vi "4 ch 8or12kHz resonance scanner (FPGA) fixed pix clock.vi"() -> ()   [LabVIEW 2012]
uses:
  <vilib>/eio/EIONode/EIONode.xnode
  <vilib>/rvi/eio/common/nirviEmuTemplateMethod_errors.vi
  <vilib>/rvi/DataTransferAndStorage/Container/XNode/niFpgaContainer.xnode
  <vilib>/platform/TimedLoop/XDataNode/XDataNode.xnode
  <vilib>/Platform/TimedLoop/XDataNode/nitl_modes.ctl
  <vilib>/Platform/TimedLoop/XDataNode/XDNodeRunTimeDep.lvlib
  <vilib>/Platform/TimedLoop/XDataNode/wakeup.ctl
  <vilib>/Platform/TimedLoop/XDataNode/timing_clust.ctl
  <vilib>/rvi/interface/RandomDataEmulation/nirviRandomDataFpgaReadWriteTemplate.vi
panel:
  in  "frequency (T:8kHz F:12kHz)":bool
  in  "lines at once":i16=4999
  in  "Start Delay (Ticks)":i16 caption="Start delay (Ticks)"
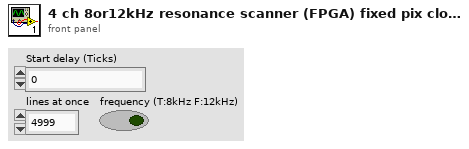
[diagram p1: front panel]
types:
  T1 = typedef "XDNodeRunTimeDep.lvlib/timing_clust.ctl" = cluster{"Expected End [f-1]":u64, "Actual End [f-1]":u64, "Finished Late? [f-1]":bool, "Expected End [i-1]":u64, "Actual End [i-1]":u64, "Finished Late? [i-1]":bool, "Expected Start [i]":u64, "Actual Start [i]":u64, "Expected Start [f]":u64, "Actual Start [f]":u64, "Source Name":string, "Structure Name":string, "Period":i64, "Deadline":i64, "Offset":i64, "Start":i64, "Priority":i32, "Timeout":i32, "Mode":T2, "Wakeup Reason":T3, "Error":errorcluster, "Source Type":string, "Secondary Source Type":string, "Global End Time":u64, "Global Start Time":u64, "Frame Duration":u64, "Iteration Duration":u64, "Assigned CPU":i32, "I/O Scan Engine Mode":u32}
  T2 = typedef "XDNodeRunTimeDep.lvlib/nitl_modes.ctl" = enum32{"No Change", "Process missed periods, maintain original phase", "Discard missed periods, maintain original phase", "Process missed periods, ignore original phase", "Discard missed periods, ignore original phase"}
  T3 = typedef "XDNodeRunTimeDep.lvlib/wakeup.ctl" = enum32{"Normal", "Aborted", "Asynchronous wakeup", "Timing source error", "Timed loop error", "Timeout"}
  T4 = cluster{"IO Module\\AI A0":i32, "IO Module\\AI A1":i32, "IO Module\\AI A3":i32, "IO Module\\AI A6":i32, "IO Module\\AI B8":i32}
  T5 = cluster{"IO Module\\AI A0":i16, "IO Module\\AI A1":i16, "IO Module\\AI A3":i16, "IO Module\\AI A6":i16, "IO Module\\AI B8":i16}
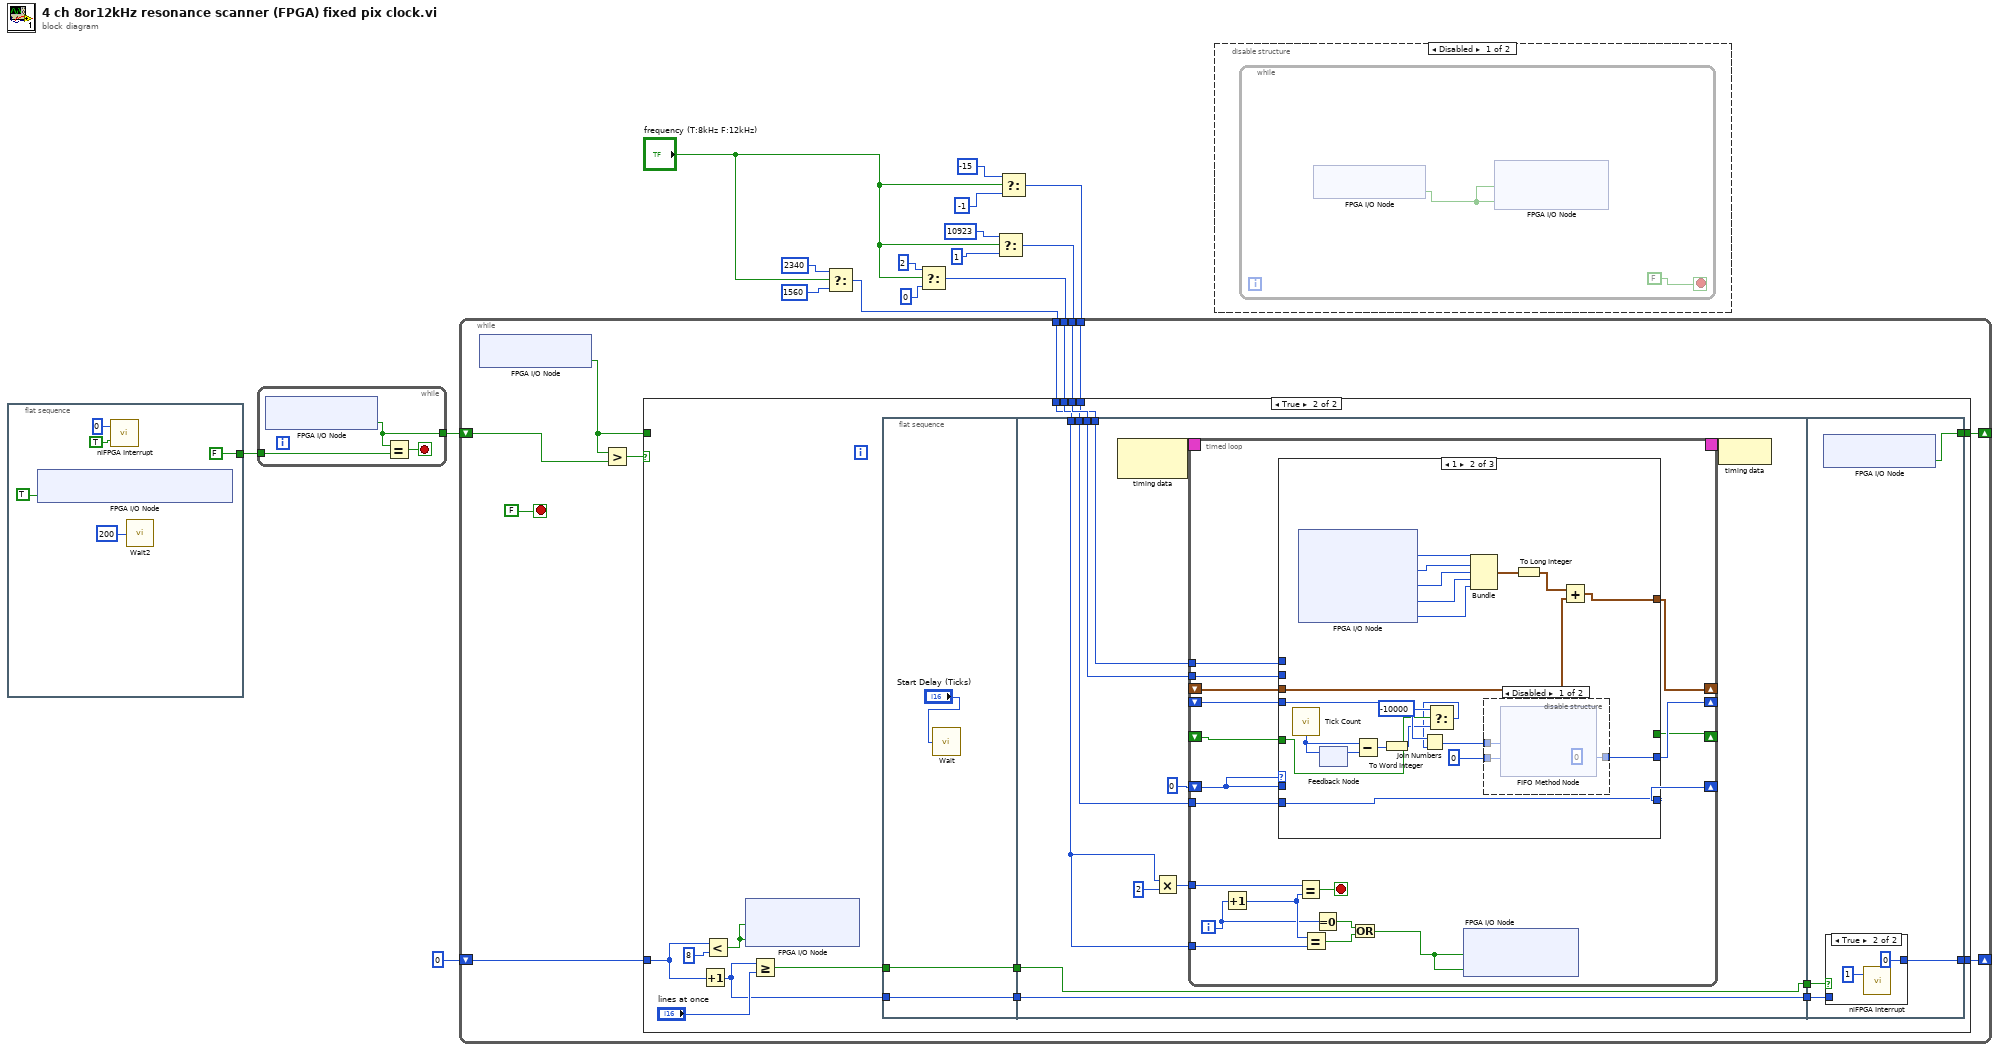
[diagram p0: block diagram]
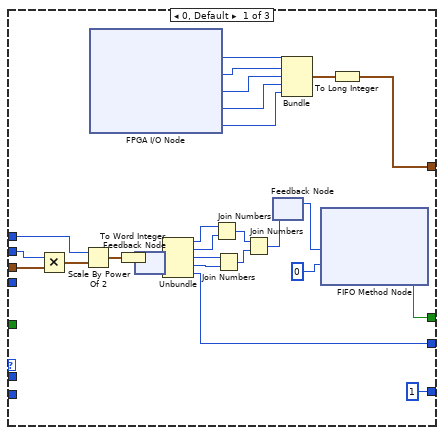
[diagram p4: hidden frame]
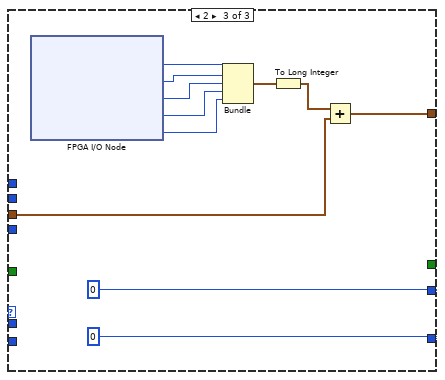
[diagram p6: hidden frame]
diagram:
  n1 = flat-sequence {
    tunnel: [FALSE ("IO Module\\DI 0")] -> w15
    frame #0 {
      n2 = xnode "FPGA I/O Node"("IO Module\\Digital Output Enable"=TRUE ("IO Module\\Digital Output Enable")) -> ()  [unwired: 1 in, 1 out]
      n3 = call <vilib>:"niFPGA Interrupt.vi"("Wait Until Cleared (F)"=TRUE, "IRQ Number (0)"=u8 0) -> ()  [unwired: 1 in]
      n4 = call "Wait2"("Count(mSec)"=u32 200) -> ()  [unwired: 1 out]
    }
  }
  n5 = while {
    tunnel: w15 -> [w24]
    tunnel: [w22] -> w14
    stop <- w23 stop-if-true
    n6 = xnode "FPGA I/O Node"() -> ("IO Module\\DI 0"=w22:bool)  [unwired: 1 in, 1 out]
    n7 = Equal?(x=w22, y=w24) -> (x = y?=w23:bool)
  }
  n8 = Select(t=i16 2340 ("samples per half period"), s="frequency (T:8kHz F:12kHz)", f=i16 1560 ("samples per half period")) -> (s? t:f=w1:i16)
  n9 = Select(t=i8 2 ("f"), s="frequency (T:8kHz F:12kHz)", f=i8 0 ("n")) -> (s? t:f=w5:i8)
  n10 = Select(t=i16 10923 ("n"), s="frequency (T:8kHz F:12kHz)", f=i16 1) -> (s? t:f=w7:i16)
  n11 = Select(t=i16 -15 ("n"), s="frequency (T:8kHz F:12kHz)", f=i16 -1 ("n")) -> (s? t:f=w6:i16)
  n12 = while {
    shift-right: [w34] -> _
    shift-left: w14 -> [w35]
    shift-right: [w32] -> _
    shift-left: i16 0 ("IRQ Number (0)") -> [w31]
    tunnel: w7 -> [w29]
    tunnel: w6 -> [w28]
    tunnel: w5 -> [w27]
    tunnel: w1 -> [w26]
    stop <- FALSE stop-if-true
    n13 = xnode "FPGA I/O Node"() -> ("IO Module\\DI 0"=w25:bool)  [unwired: 1 in, 1 out]
    n14 = Greater?(x=w25, y=w35) -> (0:w30:bool)
    n15 = case shown="True" w30 {
      tunnel: [w36 w50] -> w34
      tunnel: w31 -> [w37 w52]
      tunnel: [w37 w53] -> w32
      tunnel: w25 -> [w36 _]
      tunnel: w29 -> [_ w49]
      tunnel: w28 -> [_ w48]
      tunnel: w27 -> [_ w47]
      tunnel: w26 -> [_ w46]
      frame False {
      }
      frame True {
        n16 = Increment(x=w52) -> (x+1=w41:i16)
        n17 = Less?(x=w52, y=i16 8) -> (x < y?=w45:bool)
        n18 = xnode "FPGA I/O Node"("PXI_Trig2"=w45, "IO Module\\D0 2"=w45) -> ()  [unwired: 2 in, 2 out]
        n19 = Greater Or Equal?(x=w41, y="lines at once") -> (x >= y?=w38:bool)
        n20 = flat-sequence {
          tunnel: [w55] -> w42
          tunnel: w41 -> [w55]
          tunnel: [w54] -> w39
          tunnel: w38 -> [w54]
          tunnel: w49 -> [w62]
          tunnel: w48 -> [w61]
          tunnel: w47 -> [w60]
          tunnel: w46 -> [w59]
          tunnel: [w58] -> w43
          tunnel: w42 -> [w58]
          tunnel: [w57] -> w40
          tunnel: w39 -> [w57]
          tunnel: [w155] -> w53
          tunnel: [w154] -> w50
          tunnel: w43 -> [w153]
          tunnel: w40 -> [w152]
          frame #0 {
            n21 = call "Wait"("Count(Ticks)"="Start Delay (Ticks)") -> ()  [unwired: 1 out]
          }
          frame #1 {
            n22 = node-c288() -> (w65:T1)  [unwired: 1 in]
            n23 = Multiply(x=w59, y=i16 2) -> (x*y=w66:i16)
            n24 = timed-loop {
              tunnel: w66 -> [w85]
              timing: w65 -> [_]
              timing-out: [_] -> w64
              shift-right: [w84] -> _
              shift-left: i8 0 ("Timeout") -> [w74]
              tunnel: w59 -> [w80]
              shift-right: [w78] -> _
              shift-left: _ -> [w77]
              shift-right: [w76] -> _
              shift-left: _ -> [w75]
              tunnel: w62 -> [w73]
              tunnel: w61 -> [w72]
              tunnel: w60 -> [w71]
              shift-right: [w70] -> _
              shift-left: _ -> [w69]
              i -> [w79]
              stop <- w86 stop-if-true
              n25 = Increment(x=w79) -> (x+1=w81:i32)
              n26 = case shown="1" w74 {
                tunnel: w74 -> [_ _ _]
                tunnel: [i8 1 w113 i8 0] -> w84
                tunnel: [w106 w125 w139] -> w78
                tunnel: w77 -> [w96 w126 w140]
                tunnel: [w92 w119 i16 0 ("IO Module\\AI B8")] -> w76
                tunnel: w75 -> [_ w120 _]
                tunnel: w73 -> [w95 _ _]
                tunnel: w72 -> [w94 _ _]
                tunnel: w71 -> [_ w113 _]
                tunnel: [w90 _ _] -> w70
                tunnel: w69 -> [_ w116 _]
                frame 0, Default {
                  n27 = Multiply(x=w95, y=w96) -> (x*y=w98:T4)
                  n28 = Scale By Power Of 2(n=w94, x=w98) -> (x*2^n=w97:T4)
                  n29 = xnode "FPGA I/O Node"() -> ("IO Module\\AI A0"=w112:i16, "IO Module\\AI A1"=w111:i16, "IO Module\\AI A3"=w110:i16, "IO Module\\AI A6"=w109:i16, "IO Module\\AI B8"=w107:i16)  [unwired: 5 in, 5 out]
                  n30 = To Word Integer(number=w97) -> (16bit integer=w93:T5)
                  n31 = feedback-in #1(w93) -> ()
                  n32 = feedback #1() -> (w87:T5)  [unwired: 1 in]
                  n33 = Unbundle(w87) -> ("IO Module\\AI A0"=w102:i16, "IO Module\\AI A1"=w101:i16, "IO Module\\AI A3"=w100:i16, "IO Module\\AI A6"=w99:i16, "IO Module\\AI B8"=w92:i16)
                  n34 = Join Numbers(hi=w102, lo=w101) -> ((hi.lo)=w103:u32)
                  n35 = Join Numbers(hi=w100, lo=w99) -> ((hi.lo)=w104:u32)
                  n36 = Join Numbers(hi=w103, lo=w104) -> ((hi.lo)=w91:u64)
                  n37 = feedback-in #2(w91) -> ()
                  n38 = feedback #2() -> (w89:u64)  [unwired: 1 in]
                  n39 = Bundle("IO Module\\AI A0"=w112, "IO Module\\AI A1"=w111, "IO Module\\AI A3"=w110, "IO Module\\AI A6"=w109, "IO Module\\AI B8"=w107) -> (w108:T5)  [unwired: 1 in]
                  n40 = xnode ("FIFO Method Node")("Element"=w89, "Timeout"=0) -> ("Timed Out?"=w90:bool)  [unwired: 1 in, 1 out]
                  n41 = To Long Integer(number=w108) -> (32bit integer=w106:T4)
                }
                frame 1 {
                  n42 = call "Tick Count"() -> ("Tick Count(Ticks)"=w124:u32)
                  n43 = xnode "FPGA I/O Node"() -> ("IO Module\\AI A0"=w133:i16, "IO Module\\AI A1"=w132:i16, "IO Module\\AI A3"=w131:i16, "IO Module\\AI A6"=w130:i16, "IO Module\\AI B8"=w128:i16)  [unwired: 5 in, 5 out]
                  n44 = feedback #3() -> (w123:u32)  [unwired: 1 in]
                  n45 = feedback-in #3(w124) -> ()
                  n46 = Subtract(x=w124, y=w123) -> (x-y=w122:u32)
                  n47 = To Word Integer(number=w122) -> (16bit integer=w117:i16)
                  n48 = Select(t=i16 -10000, s=w116, f=w117) -> (s? t:f=w114:i16)
                  n49 = Join Numbers(hi=w120, lo=w114) -> ((hi.lo)=w118:u32)
                  n50 = Bundle("IO Module\\AI A0"=w133, "IO Module\\AI A1"=w132, "IO Module\\AI A3"=w131, "IO Module\\AI A6"=w130, "IO Module\\AI B8"=w128) -> (w129:T5)  [unwired: 1 in]
                  n51 = disable-structure shown="Disabled" {
                    disable-tunnel: 0 ("Timeout") -> [w136 _]
                    disable-tunnel: [i16 0 ("IO Module\\AI B8") _] -> w119
                    disable-tunnel: w118 -> [w134 _]
                    frame Disabled {
                      n52 = xnode ("FIFO Method Node")("Element"=w134, "Timeout"=w136) -> ()  [unwired: 1 in, 2 out]
                    }
                    frame Enabled {
                    }
                  }
                  n53 = To Long Integer(number=w129) -> (32bit integer=w127:T4)
                  n54 = Add(x=w127, y=w126) -> (x+y=w125:T4)
                }
                frame 2 {
                  n55 = xnode "FPGA I/O Node"() -> ("IO Module\\AI A0"=w147:i16, "IO Module\\AI A1"=w146:i16, "IO Module\\AI A3"=w145:i16, "IO Module\\AI A6"=w144:i16, "IO Module\\AI B8"=w142:i16)  [unwired: 5 in, 5 out]
                  n56 = Bundle("IO Module\\AI A0"=w147, "IO Module\\AI A1"=w146, "IO Module\\AI A3"=w145, "IO Module\\AI A6"=w144, "IO Module\\AI B8"=w142) -> (w143:T5)  [unwired: 1 in]
                  n57 = To Long Integer(number=w143) -> (32bit integer=w141:T4)
                  n58 = Add(x=w141, y=w140) -> (x+y=w139:T4)
                }
              }
              n59 = Equal?(x=w85, y=w81) -> (x = y?=w86:bool)
              n60 = Equal?(x=w81, y=w80) -> (x = y?=w82:bool)
              n61 = Equal To 0?(x=w79) -> (x = 0?=w83:bool)
              n62 = Or(x=w83, y=w82) -> (x .or. y?=w68:bool)
              n63 = xnode "FPGA I/O Node"("IO Module\\D0 1"=w68, "PXI_Trig1"=w68) -> ()  [unwired: 2 in, 2 out]
            }
            n64 = node-c288(w64) -> ()
          }
          frame #2 {
            n65 = xnode "FPGA I/O Node"() -> ("IO Module\\DI 0"=w154:bool)  [unwired: 1 in, 1 out]
            n66 = case shown="True" w152 {
              tunnel: w153 -> [w156 _]
              tunnel: [w156 u8 0] -> w155
              frame False {
              }
              frame True {
                n67 = call <vilib>:"niFPGA Interrupt.vi"("IRQ Number (0)"=u8 1) -> ()  [unwired: 2 in]
              }
            }
          }
        }
      }
    }
  }
  n68 = disable-structure shown="Disabled" {
    frame Disabled {
      n69 = while {
        stop <- FALSE stop-if-true
        n70 = xnode "FPGA I/O Node"() -> ("IO Module\\DI 0"=w160:bool)  [unwired: 1 in, 1 out]
        n71 = xnode "FPGA I/O Node"("IO Module\\D0 3"=w160, "PXI_Trig3"=w160) -> ()  [unwired: 2 in, 2 out]
      }
    }
    frame Enabled {
    }
  }
